vi "Get Column Data Types.vi"(11 "DataGrid Config":refnum<class "DataGrid Config.lvclass">) -> (3 "Column Data Type Names":string[][](array[string]))   [LabVIEW 2018, in "DataGrid Config.lvclass"]
uses:
  DataGrid Config.lvclass
  DataGrid Config.lvclass/DataGrid Config.ctl
  Data Type Classes/Generic/Generic Data Type.lvclass
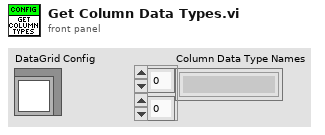
[diagram p1: front panel]
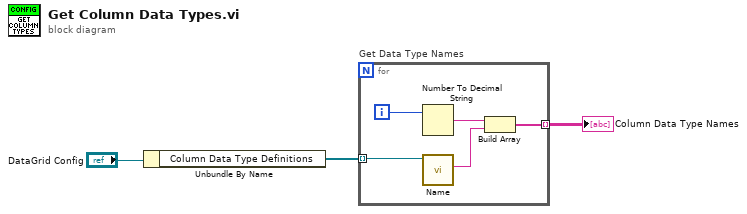
[diagram p0: block diagram]
diagram:
  n1 = Unbundle By Name("DataGrid Config") -> ("Column Data Type Definitions"=w1:refnum<class "Generic Data Type.lvclass">[])
  n2 = for "Get Data Type Names" {
    tunnel: w1 -> [w8] mode=indexing
    tunnel: [w4] -> w3 mode=indexing
    i -> [w7]
    n3 = Number To Decimal String(number=w7) -> (decimal integer string=w6:string)  [unwired: 1 in]
    n4 = call-dynamic "Name.vi"("Generic Data Type in"=w8) -> ("String"=w5:string)  [unwired: 9 in, 1 out]
    n5 = Build Array(w6, w5) -> (w4:string[])
  }
  "Column Data Type Names" <- w3
